vi "AdvancedVIMTools.vi"   [LabVIEW 2017]
uses:
  a8b993a6-bd4b-48f8-be96-b70c68c7776b.vi
panel:
  # "More advanced tools can be used for type parsing.\n\nIn the future, additional \"Type Algebra\" will be added to LabVIEW. No date was given!"
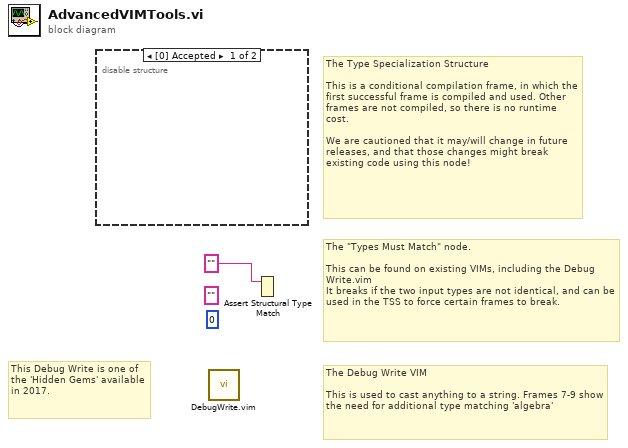
[diagram p0: block diagram]
diagram:
  (unwired) 0
  (unwired) ""
  # "This Debug Write is one of the 'Hidden Gems' available in 2017."
  # "The Debug Write VIM\n\nThis is used to cast anything to a string. Frames 7-9 show the need for additional type matching 'algebra'"
  # "The \"Types Must Match\" node.\n\nThis can be found on existing VIMs, including the Debug Write.vim\nIt breaks if the two input types are not identical, and can be used in the TSS to force certain frames to break."
  # "The Type Specialization Structure\n\nThis is a conditional compilation frame, in which the first successful frame is compiled and used. Other frames are not compiled, so there is no runtime cost.\n\nWe are cautioned that it may/will change in future releases, and that those changes might break existing code using this node!"
  n1 = disable-structure shown="[0] Accepted" {
    frame Enabled {
      # "Unbroken for 1D arrays"
    }
    frame Disabled {
      # "Unbroken for scalars"
    }
  }
  n2 = call "DebugWrite.vim"() -> ()  [unwired: 11 in, 1 out]
  n3 = Assert Structural Type Match(1:"") -> ()  [unwired: 1 in]
